vi "Read.vi"(8 "error in (no error)":errorcluster, 11 "Event Command Config in":refnum<class "Event Command Config.lvclass">) -> (0 "error out":errorcluster, 2 "Message":string, 3 "Event Command Config out":refnum<class "Event Command Config.lvclass">)   [LabVIEW 2020, in "VolatusSeqConfig.lvlib" / "Event Command Config.lvclass"]
uses:
  Event Command Config.lvclass
  Event Command Config.lvclass/Event Command Config.ctl
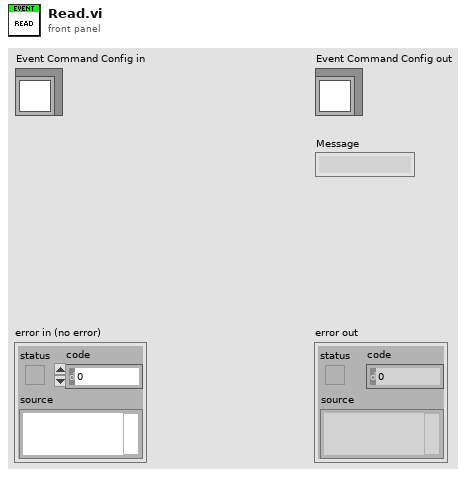
[diagram p1: front panel]
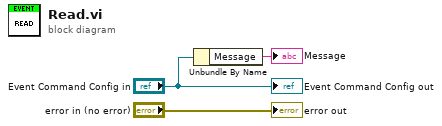
[diagram p0: block diagram]
diagram:
  n1 = Unbundle By Name("Event Command Config in") -> ("Message"=→"Message":string)
  "error out" <- "error in (no error)"
  "Event Command Config out" <- "Event Command Config in"
